vi "uintComparisons.vi"(8 "Error in (no error)":errorcluster, 10 "Int2 in":refnum<class "UintClass.lvclass">, 11 "Int1 in":refnum<class "UintClass.lvclass">) -> (0 "Error out":errorcluster, 1 "Timing":u32, 2 "Uint1 != Uint2?":bool, 3 "Uint1 = Uint2?":bool, 4 "Uint1 >= Uint2?":bool, 5 "Uint1 > Uint2?":bool, 6 "Uint1 <= Uint2?":bool, 7 "Uint1 < Uint2?":bool)   [LabVIEW 2011, in "UintClass.lvclass"]
uses:
  UintClass.lvclass
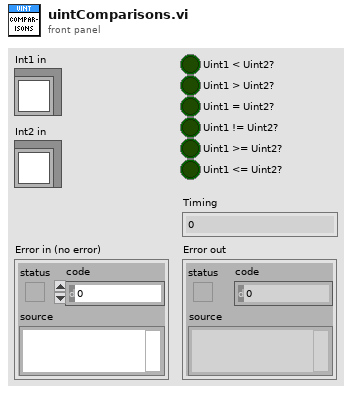
[diagram p1: front panel]
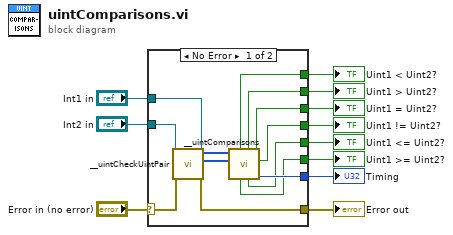
[diagram p0: block diagram]
diagram:
  n1 = case shown="No Error" "Error in (no error)" {
    selector: "Error in (no error)" -> [w22 w25]
    tunnel: "Int1 in" -> [w24 _]
    tunnel: "Int2 in" -> [w23 _]
    tunnel: [w21 w25] -> w8
    tunnel: [w18 _] -> w7
    tunnel: [w17 _] -> w6
    tunnel: [w16 _] -> w5
    tunnel: [w15 _] -> w4
    tunnel: [w14 _] -> w3
    tunnel: [w13 _] -> w2
    tunnel: [w12 _] -> w1
    frame No Error {
      n2 = call "__uintCheckUintPair.vi"("Error in (no error)"=w22, "Uint2 in"=w23, "Uint1 in"=w24) -> ("Error out"=w21:errorcluster, "Uint2 out"=w19:u8[], "Uint1 out"=w20:u8[])  [unwired: 5 in, 1 out]
      n3 = call "__uintComparisons.vi"("Uint2 in"=w19, "Uint1 in"=w20) -> ("Timing comparison"=w18:u32, "Uint1 != Uint2"=w14:bool, "Uint1 = Uint2"=w15:bool, "Uint1 <= Uint2"=w12:bool, "Uint1 > Uint2"=w16:bool, "Uint1 >= Uint2"=w13:bool, "Uint1 < Uint2"=w17:bool)  [unwired: 3 in]
    }
    frame Error {
    }
  }
  "Error out" <- w8
  "Timing" <- w7
  "Uint1 < Uint2?" <- w6
  "Uint1 > Uint2?" <- w5
  "Uint1 = Uint2?" <- w4
  "Uint1 != Uint2?" <- w3
  "Uint1 <= Uint2?" <- w1
  "Uint1 >= Uint2?" <- w2
